vi "Get UIDs.vi"(8 "error in":errorcluster, 10 "Class Name":T1, 11 "VI Refnum In":refnum<vi>) -> (0 "error out":errorcluster, 2 "UIDs":i32[](array[numeric]), 3 "VI Refnum Out":refnum<vi>)   [LabVIEW 2020]
doc: "Retrieve UIDs of specified class from the active VI."
uses:
  src/Type Definitions/Class Name--enum.ctl
  <vilib>/Utility/traverseref.llb/TRef TravTarget.ctl
  <vilib>/Utility/traverseref.llb/VI Scripting - Traverse.lvlib
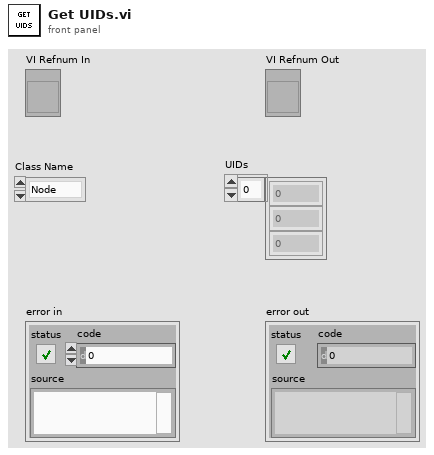
[diagram p1: front panel]
types:
  T1 = typedef "Class Name--enum.ctl" = enum16{"Node", "Wire"}
  T2 = typedef "TRef TravTarget.ctl" = enum16{"FP", "BD", "Other"}
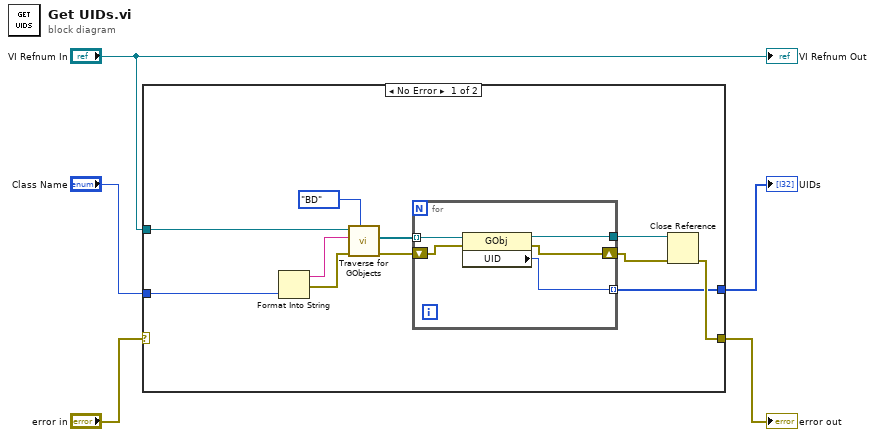
[diagram p0: block diagram]
diagram:
  n1 = case shown="No Error" "error in" {
    selector: "error in" -> [_ w22]
    tunnel: "Class Name" -> [w8 _]
    tunnel: [w13 w22] -> w4
    tunnel: [w7 _] -> w2
    tunnel: "VI Refnum In" -> [w6 _]
    frame No Error {
      n2 = Format Into String(w8) -> (resulting string=w12:string, error out=w16:errorcluster)  [unwired: 3 in]
      n3 = call <vilib>:"Traverse for GObjects.vi"("Traverse Target"=TRef_TravTarget."BD", "error in (no error)"=w16, "Class Name"=w12, "VI Refnum"=w6) -> ("error out"=w15:errorcluster, "References"=w11:refnum<vi>[])  [unwired: 4 in, 2 out]
      n4 = for {
        tunnel: w11 -> [w19] mode=indexing
        tunnel: [w18] -> w10
        shift-right: [w20] -> w14
        shift-left: w15 -> [w21]
        tunnel: [w17] -> w7 mode=indexing
        n5 = property class="GObj"(reference=w19, error in=w21) -> (reference out=w18:refnum<vi>, error out=w20:errorcluster, "UID"=w17:i32)
      }
      n6 = Close Reference(reference=w10, error in (no error)=w14) -> (error out=w13:errorcluster)
    }
    frame Error {
      # "Pass error without further action"
    }
  }
  "error out" <- w4
  "UIDs" <- w2
  "VI Refnum Out" <- "VI Refnum In"
